vi "Reserve Sessions Wrapper.vi"(8 "error in":errorcluster, 11 "request data":T8) -> (0 "error out":errorcluster, 3 "response data":T1)   [LabVIEW 2020, in "Plug-In SDK Session Management V1 API.lvlib" / "Session Reservation.lvclass"]
uses:
  Session Reservation.lvclass
  gRPC/Generated APIs/ni/measurementlink/sessionmanagement/v1/RPC Messages/ni_measurementlink_sessionmanagement_v1_ReserveSessionsRequest.ctl
  gRPC/Generated APIs/ni/measurementlink/sessionmanagement/v1/RPC Messages/ni_measurementlink_PinMapContext.ctl
  gRPC/Generated APIs/ni/measurementlink/sessionmanagement/v1/RPC Messages/ni_measurementlink_sessionmanagement_v1_ReserveSessionsResponse.ctl
  gRPC/Generated APIs/ni/measurementlink/sessionmanagement/v1/RPC Messages/ni_measurementlink_sessionmanagement_v1_SessionInformation.ctl
  gRPC/Generated APIs/ni/measurementlink/sessionmanagement/v1/RPC Messages/nidevice_grpc_Session.ctl
  gRPC/Generated APIs/ni/measurementlink/sessionmanagement/v1/RPC Messages/ni_measurementlink_sessionmanagement_v1_ChannelMapping.ctl
  gRPC/Generated APIs/ni/measurementlink/sessionmanagement/v1/RPC Messages/ni_measurementlink_sessionmanagement_v1_MultiplexerSessionInformation.ctl
  gRPC/Generated APIs/ni/measurementlink/sessionmanagement/v1/RPC Messages/ni_measurementlink_sessionmanagement_v1_ReserveSessionsResponse_GroupMappingsEntry.ctl
  gRPC/Generated APIs/ni/measurementlink/sessionmanagement/v1/RPC Messages/ni_measurementlink_sessionmanagement_v1_ResolvedPinsOrRelays.ctl
  Discovery V1/TypeDefs/gRPC Client Cache FGV Action.ctl
  gRPC/Generated APIs/ni/measurementlink/sessionmanagement/v1/ni.measurementlink.sessionmanagement.v1.api.lvlib
  Discovery V1/Plug-In SDK Discovery V1 API.lvlib
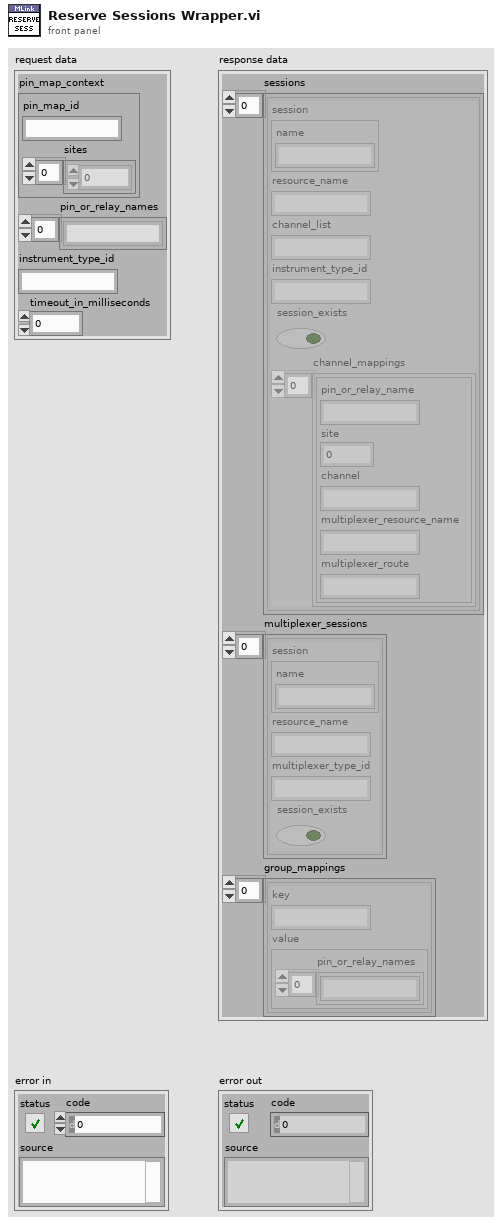
[diagram p1: front panel]
types:
  T1 = typedef "ni.measurementlink.sessionmanagement.v1.api.lvlib/ni_measurementlink_sessionmanagement_v1_ReserveSessionsResponse.ctl" = cluster{"sessions":T2[], "multiplexer_sessions":T5[], "group_mappings":T6[]}
  T2 = typedef "ni.measurementlink.sessionmanagement.v1.api.lvlib/ni_measurementlink_sessionmanagement_v1_SessionInformation.ctl" = cluster{"session":T3, "resource_name":string, "channel_list":string, "instrument_type_id":string, "session_exists":bool, "channel_mappings":T4[]}
  T3 = typedef "ni.measurementlink.sessionmanagement.v1.api.lvlib/nidevice_grpc_Session.ctl" = cluster{"name":string}
  T4 = typedef "ni.measurementlink.sessionmanagement.v1.api.lvlib/ni_measurementlink_sessionmanagement_v1_ChannelMapping.ctl" = cluster{"pin_or_relay_name":string, "site":i32, "channel":string, "multiplexer_resource_name":string, "multiplexer_route":string}
  T5 = typedef "ni.measurementlink.sessionmanagement.v1.api.lvlib/ni_measurementlink_sessionmanagement_v1_MultiplexerSessionInformation.ctl" = cluster{"session":T3, "resource_name":string, "multiplexer_type_id":string, "session_exists":bool}
  T6 = typedef "ni.measurementlink.sessionmanagement.v1.api.lvlib/ni_measurementlink_sessionmanagement_v1_ReserveSessionsResponse_GroupMappingsEntry.ctl" = cluster{"key":string, "value":T7}
  T7 = typedef "ni.measurementlink.sessionmanagement.v1.api.lvlib/ni_measurementlink_sessionmanagement_v1_ResolvedPinsOrRelays.ctl" = cluster{"pin_or_relay_names":string[]}
  T8 = typedef "ni.measurementlink.sessionmanagement.v1.api.lvlib/ni_measurementlink_sessionmanagement_v1_ReserveSessionsRequest.ctl" = cluster{"pin_map_context":T9, "pin_or_relay_names":string[], "instrument_type_id":string, "timeout_in_milliseconds":i32}
  T9 = typedef "ni.measurementlink.sessionmanagement.v1.api.lvlib/ni_measurementlink_PinMapContext.ctl" = cluster{"pin_map_id":string, "sites":i32[]}
  T10 = typedef "Plug-In SDK Discovery V1 API.lvlib/gRPC Client Cache FGV Action.ctl" = enum16{"Get Client", "Recreate Client", "Destroy Client", "Update ClusterId"}
  T11 = typedef "grpc-lvsupport-release.lvlib/grpcId.ctl" = u64
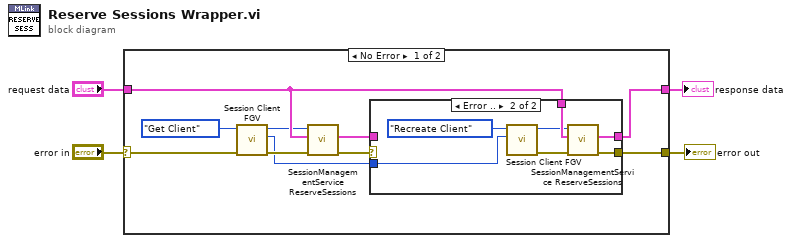
[diagram p0: block diagram]
diagram:
  n1 = case shown="No Error" "error in" {
    selector: "error in" -> [w14 w24]
    tunnel: "request data" -> [w7 _]
    tunnel: [w9 _] -> w3
    tunnel: [w11 w24] -> w1
    frame No Error {
      n2 = call "Session Client FGV.vi"("error in"=w14, "action"=gRPC_Client_Cache_FGV_Action."Get Client") -> ("error out"=w13:errorcluster, "unique id out"=w5:u64, "grpc client id"=w6:T11)  [unwired: 7 in]
      n3 = call "SessionManagementService ReserveSessions.vi"("error in"=w13, "Request Data"=w7, "gRPC ID"=w6) -> ("error out"=w12:errorcluster, "Response Data"=w8:T1)  [unwired: 6 in, 1 out]
      n4 = case shown="Error .." w12 {
        selector: w12 -> [w16 _]
        tunnel: [w16 w22] -> w11
        tunnel: [w15 w21] -> w9
        tunnel: w8 -> [w15 _]
        tunnel: w5 -> [_ w18]
        tunnel: w7 -> [_ w20]
        frame No Error {
        }
        frame Error {
          n5 = call "Session Client FGV.vi"("unique id in"=w18, "action"=gRPC_Client_Cache_FGV_Action."Recreate Client") -> ("error out"=w23:errorcluster, "grpc client id"=w17:T11)  [unwired: 7 in, 1 out]
          n6 = call "SessionManagementService ReserveSessions.vi"("error in"=w23, "Request Data"=w20, "gRPC ID"=w17) -> ("error out"=w22:errorcluster, "Response Data"=w21:T1)  [unwired: 6 in, 1 out]
        }
      }
    }
    frame Error {
    }
  }
  "error out" <- w1
  "response data" <- w3
